vi "Calibration Dialog.vi"(11 "HAL Config Data in":T1) -> (3 "HAL Config Data out":T1)   [LabVIEW 2014]
uses:
  TypeDefs/HAL Config Data.ctl
panel:
  in  "Gain":sgl[][](array[numeric])=[[1.0, 1.0, 1.0, 1.0], [1.0, 1.0, 1.0, 1.0], [1.0, 1.0, 1.0, 1.0], [1.0, 1.0, 1.0, 1.0]]
  in  "Offset":sgl[][](array[numeric])=[[0.0, 0.0, 0.0, 0.0], [0.0, 0.0, 0.0, 0.0], [0.0, 0.0, 0.0, 0.0], [0.0, 0.0, 0.0, 0.0]]
  in  "Channel List 4":bool[](array[boolean])=[FALSE, FALSE, FALSE, FALSE]
  in  "Channel List 3":bool[](array[boolean])=[FALSE, FALSE, FALSE, FALSE]
  in  "Channel List 2":bool[](array[boolean])=[FALSE, FALSE, FALSE, FALSE]
  in  "Channel List 1":bool[](array[boolean])=[FALSE, FALSE, FALSE, FALSE]
  in  "Cancel":bool
  in  "OK":bool
  # "Selección de Transductores"
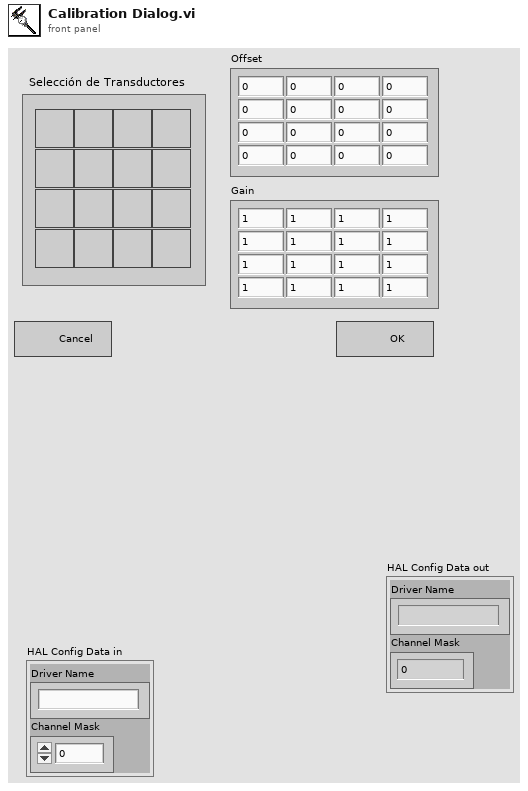
[diagram p1: front panel]
types:
  T1 = typedef "HAL Config Data.ctl" = cluster{"Driver Name":string, "Channel Mask":u64}
  T2 = typedef "HAL Config Data.ctl" = cluster{"Driver Name":string, "Channel Mask":u64, "Offset":sgl[], "Gain":sgl[]}
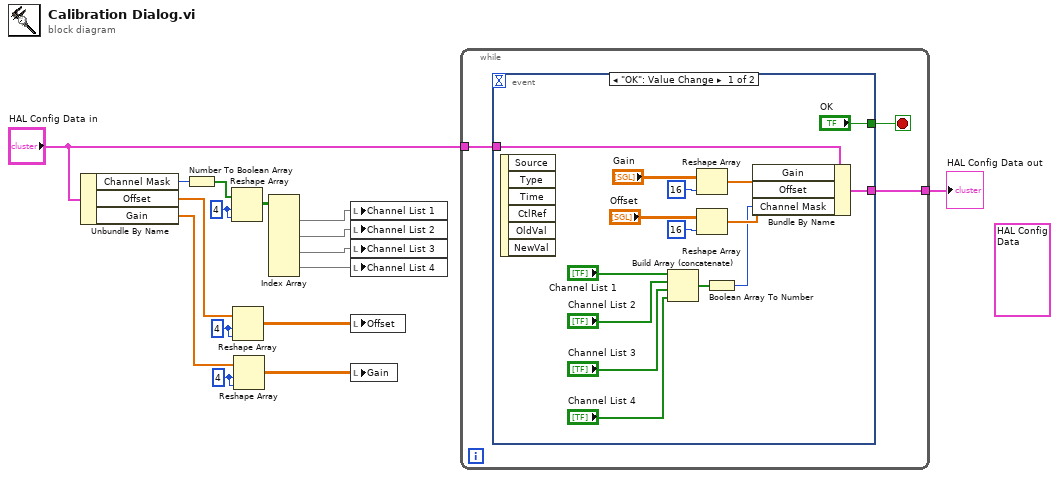
[diagram p0: block diagram]
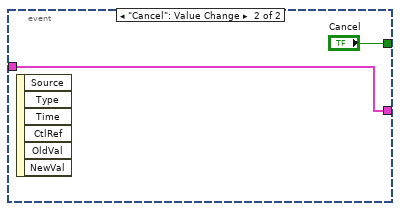
[diagram p2: hidden frame]
diagram:
  (unwired) T2 {"Driver Name"="", "Channel Mask"=1, "Offset"=[0.0, 0.0, 0.0, 0.0, 0.0, 0.0, 0.0, 0.0, 0.0, 0.0, 0.0, 0.0, 0.0, 0.0, 0.0, 0.0], "Gain"=[1.0, 1.0, 1.0, 1.0, 1.0, 1.0, 1.0, 1.0, 1.0, 1.0, 1.0, 1.0, 1.0, 1.0, 1.0, 1.0]} ("HAL Config Data out")
  w3 = 4 ("dimension size")
  w5 = 4 ("dimension size")
  w13 = 4 ("dimension size")
  n1 = Unbundle By Name("HAL Config Data in") -> ("Channel Mask"=w14:u64, "Offset"=w6:sgl[], "Gain"=w1:sgl[])
  n2 = Number To Boolean Array(number=w14) -> (Boolean array=w12:bool[])
  n3 = Reshape Array(w12, w13, w13) -> (w11:bool[][])
  n4 = Reshape Array(w6, w5, w5) -> (w4:sgl[][])
  n5 = Reshape Array(w1, w3, w3) -> (w2:sgl[][])
  n6 = Index Array(array=w11) -> (element #1=w10:bool[], element #2=w9:bool[], element #3=w8:bool[], element #4=w7:bool[])  [unwired: 8 in]
  n7 = local write "Channel List 1"(w10) -> ()
  n8 = local write "Channel List 2"(w9) -> ()
  n9 = local write "Channel List 3"(w8) -> ()
  n10 = local write "Channel List 4"(w7) -> ()
  n11 = local write "Offset"(w4) -> ()
  n12 = local write "Gain"(w2) -> ()
  n13 = while {
    tunnel: "HAL Config Data in" -> [w18]
    tunnel: [w19] -> w16
    stop <- w17 stop-if-true
    n14 = event shown="[0] \"OK\": Value Change" {
      selector: _ -> [_ _]
      dyn-events: _ -> [_ _]
      timeout: _ -> [_ _]
      tunnel: [w34 w36] -> w19
      tunnel: w18 -> [w33 w36]
      tunnel: ["OK" "Cancel"] -> w17
      event "OK": Value Change {
        n15 = event-data() -> ()  [unwired: 1 in, 6 out]
        n16 = Build Array (concatenate)("Channel List 1", "Channel List 2", "Channel List 3", "Channel List 4") -> (w32:bool[])
        n17 = Reshape Array("Gain", 16 ("dimension size")) -> (w23:sgl[])
        n18 = Reshape Array("Offset", 16 ("dimension size")) -> (w22:sgl[])
        n19 = Boolean Array To Number(Boolean array=w32) -> (number=w21:u32)
        n20 = Bundle By Name(cluster=w33, "Gain"=w23, "Offset"=w22, "Channel Mask"=w21) -> (w34:T1)
      }
      event "Cancel": Value Change {
        n21 = event-data() -> ()  [unwired: 1 in, 6 out]
      }
    }
  }
  "HAL Config Data out" <- w16
